vi "SVFA Power Spectrum (N Ch).vi"(0 "scaled signals [EU]":waveform(dbl)[](array[waveform]), 2 "window":T8=1 items=["None"=0, "Hanning"=1, "Hamming"=2, "Blackman-Harris"=3, "Exact Blackman"=4, "Blackman"=5, "Flat Top"=6, "4 Term B-Harris "=7, "7 Term B-Harris"=8, "Low Sidelobe"=9, "Force"=64, "Exponential"=65, "Blackman Nuttall"=11, "Triangle"=30, "Bartlett-Hanning"=31, "Bohman"=32, "Parzen"=33, "Welch"=34, "Kaiser"=60, "Dolph-Chebyshev"=61, "Gaussian"=62], 4 "dB On (T)":bool=TRUE, 5 "error in (no error)":errorcluster, 7 "averaging parameters":T7={"averaging mode"=enum."No averaging", "weighting mode"=enum."Exponential", "number of averages"=10, "linear mode"=enum."One shot"}, 9 "restart averaging (F)":bool) -> (11 "averaging done":bool, 13 "averages completed":dbl, 14 "power spectra [dB EU]":cluster{"f0":dbl, "df":dbl, "magnitude":dbl[]}[](array[cluster]) {"magnitude" format="%.2p"; "df" format="%.2p"; "f0" format="%.2p"}, 15 "unit labels":string[](array[string]), 18 "spectrum info":T1[](array[typedef]) {"x-axis units" items=["Time (s)"=0, "Frequency-CB (Hz)"=1, "Frequency-CPB (Hz)"=1248, "Frequency-Arbitrary (Hz)"=2357, "Quefrency (s)"=2, "Revolutions (rev)"=3, "Order"=4, "Speed (RPM)"=11, "Speed (rad/s)"=21, "Index"=65535]; "weighting filter" items=["Linear", "A-weighting", "B-weighting", "C-weighting", "ITU-R 468-4", "Dolby", "CCITT", "C-message", "Wb", "Wc", "Wd", "We", "Wf", "Wh", "Wj", "Wk", "Wm", "AES17 20 kHz lowpass", "AES17 40 kHz lowpass", "AES17 20 kHz highpass", "AES17 40 kHz highpass"]; "dB reference [EU]" format="%.2f"; "engineering units" items=["custom..."=0, "V"=1, "A"=21, "C"=30, "pC"=31, "s"=32, "-"=29, "Pa"=2, "N"=20, "g"=3, "m/s^2"=4, "m/s"=5, "m"=6, "mm/s"=12, "mm"=13, "micron/s"=14, "micron"=15, "in/s^2"=7, "in/s"=8, "in"=9, "mil/s"=10, "mil"=11, "rad/s^2"=16, "rad/s"=17, "rad"=18, "deg/s^2"=26, "deg/s"=27, "deg"=28, "RPM"=22, "cycle/s^2"=23, "Hz"=24, "cycle"=25, "strain"=19]; "spectral info"."window" items=["None "=0, "Hanning"=1, "Hamming"=2, "Blackman-Harris"=3, "Exact Blackman"=4, "Blackman"=5, "Flat Top"=6, "4 Term B-Harris "=7, "7 Term B-Harris"=8, "Low Sidelobe"=9, "Force - Exponential"=10, "Gaussian"=62]}, 19 "error out":errorcluster)   [LabVIEW 2017]
doc: "Computes the power spectrum of <B>scaled signal [EU]</B>. Use the power spectrum to quantify signal components as a function of frequency. Wire data to the <B>scaled signal [EU]</B> input to determine the polymorphic instance to use or manually select the instance."
uses:
  <vilib>/addons/_NISVFA/_Shared subVIs/Controls/svc_Window.ctl
  <vilib>/addons/_NISVFA/_Shared subVIs/Controls/svc_Spectrum Info.ctl
  <vilib>/addons/_NISVFA/_Shared subVIs/Controls/svc_X-Axis Units.ctl
  <vilib>/addons/_NISVFA/_Shared subVIs/Controls/svc_Spectrum Type.ctl
  <vilib>/addons/_NISVFA/_Shared subVIs/Controls/svc_Engineering Units Text Ring.ctl
  <vilib>/addons/_NISVFA/_Shared subVIs/Controls/svc_Weighting Filter Text Ring.ctl
  <vilib>/addons/_NISVFA/_Shared subVIs/Controls/svc_Complimentary Spectrum Units.ctl
  <vilib>/Analysis/2dsp.llb/Power Spectrum (DBL).vi
  <vilib>/Analysis/2dsp.llb/Real FFT.vi
  <vilib>/addons/_NISVFA/_Shared subVIs/Spectrum Averaging/svfa_No Average Array (complex).vi
  <vilib>/Analysis/4window.llb/Force Window.vi
  <vilib>/Analysis/4window.llb/Force Window (DBL).vi
  <vilib>/Analysis/4window.llb/Exponential Window.vi
  <vilib>/Analysis/4window.llb/Exponential Window (DBL).vi
  <vilib>/addons/_NISVFA/_Shared subVIs/Common/svc_Get Weighting Enum and Labels.vi
  <vilib>/addons/_NISVFA/_Shared subVIs/Common/svc_Unit Label Lexical Class.vi
  <vilib>/addons/_NISVFA/_Shared subVIs/Common/svc_Engineering Units to Unit Label.vi
  <vilib>/addons/_NISVFA/_Shared subVIs/Common/svc_Format Value (DBL).vi
  <vilib>/Utility/error.llb/Error Cluster From Error Code.vi
  <vilib>/Analysis/0measdsp.llb/Scaled Time Domain Window.vi
  <vilib>/Analysis/0measdsp.llb/Scaled Time Domain Window (DBL).vi
  <vilib>/addons/_NISVFA/_Spectrum Processing/subVIs/svfa_Spectrum Info Window to windowTd Type Def.vi
  <vilib>/addons/_NISVFA/_Shared subVIs/Common/svc_Unit Label to Engineering Units.vi
  <vilib>/addons/_NISVFA/_Shared subVIs/Common/svc_Window Parameters.vi
  <vilib>/addons/_NISVFA/_Shared subVIs/Common/svc_Get Window Info.vi
  <vilib>/Analysis/NI_AALPro.lvlib
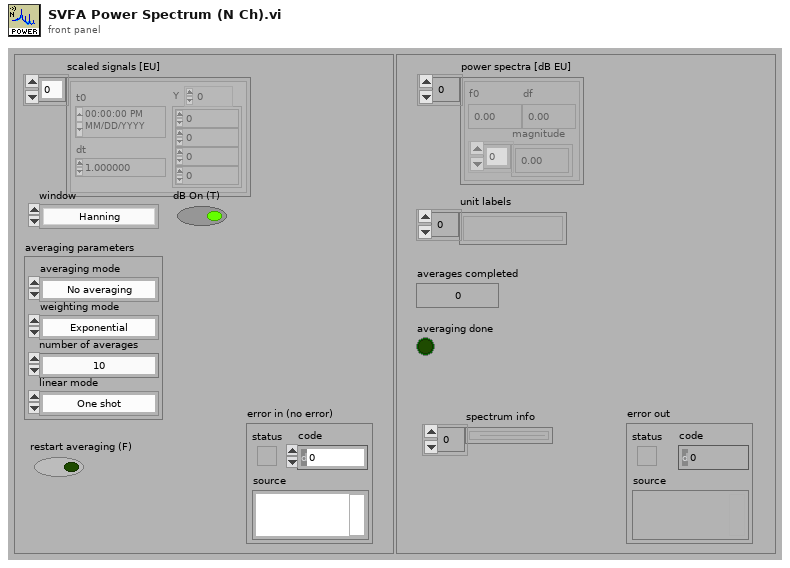
[diagram p1: front panel]
types:
  T1 = typedef "svc_Spectrum Info.ctl" = cluster{"channel name":string, "description":string, "x-axis units":T2, "spectral info":cluster{"spectrum type":T3, "linear/dB":enum16{"linear", "dB"}, "window":u16, "window size":i32, "FFT size":i32}, "engineering units":T4, "custom label":string, "dB reference [EU]":dbl, "peak units":enum16{"rms", "peak", "peak-peak"}, "weighting filter":T5, "spectral density?":bool, "unit label":string, "spectrum skewed?":bool, "complimentary spectrum units":T6}
  T2 = typedef "svc_X-Axis Units.ctl" = u16
  T3 = typedef "svc_Spectrum Type.ctl" = enum16{"FFT Spectrum [complex]", "Amplitude [Magnitude]", "Power [Magnitude^2]", "Cross Spectrum [complex]", "Frequency Response [Complex]"}
  T4 = typedef "svc_Engineering Units Text Ring.ctl" = u16
  T5 = typedef "svc_Weighting Filter Text Ring.ctl" = u16
  T6 = typedef "svc_Complimentary Spectrum Units.ctl" = enum16{"none", "radians", "degrees", "cycles", "imaginary"}
  T7 = cluster{"averaging mode":enum16{"No averaging", "Vector averaging", "RMS averaging", "Peak hold"}, "weighting mode":enum16{"Linear", "Exponential"}, "number of averages":u32, "linear mode":enum16{"One shot", "Auto restart"}}
  T8 = typedef "svc_Window.ctl" = u32
  T9 = enum16{"Restart processing", "Continue processing", "Skip processing"}
  T10 = cluster{"complex FFT":cdb[], "real FFT":dbl[], "f0":dbl, "df":dbl, "averages completed":dbl, "averaging parameters":cluster{"averaging mode":enum16{"No averaging", "Vector averaging", "RMS averaging", "Peak hold"}, "weighting mode":enum16{"Linear", "Exponential"}, "number of averages":u32, "linear mode":enum16{"One shot", "Auto restart"}}}
  T11 = cluster{"spectrum type":T3, "linear/dB":enum16{"linear", "dB"}, "window":u16, "window size":i32, "FFT size":i32}
  T12 = cluster{"complex FFT":cdb[], "real FFT":dbl[], "f0":dbl, "df":dbl, "averages completed":dbl, "averaging parameters":cluster{"averaging mode":enum16{"No averaging", "Vector averaging", "RMS averaging", "Peak hold"}, "weighting mode":enum16{"Linear", "Exponential"}, "number of averages":u32, "linear mode":enum16{"One shot", "Auto restart"}}}[]
  T13 = cluster{"complex FFT":cdb[], "Mag/Real FFT":dbl[], "f0":dbl, "df":dbl, "averages completed":dbl, "averaging parameters":cluster{"averaging mode":enum16{"No averaging", "Vector averaging", "RMS averaging", "Peak hold"}, "weighting mode":enum16{"Linear", "Exponential"}, "number of averages":u32, "linear mode":enum16{"One shot", "Auto restart"}}}[]
  T14 = enum16{"No averaging", "Vector averaging", "RMS averaging", "Peak hold"}
  T15 = typedef "svc_Channel Info.ctl" = cluster{"sensor sensitivity":dbl, "engineering units":T4, "dB reference":dbl, "custom label":string, "weighting filter":T5, "pregain":dbl}
  T16 = cluster{"complex FFT":cdb[], "Mag/Real FFT":dbl[], "f0":dbl, "df":dbl, "averages completed":dbl, "averaging parameters":cluster{"averaging mode":enum16{"No averaging", "Vector averaging", "RMS averaging", "Peak hold"}, "weighting mode":enum16{"Linear", "Exponential"}, "number of averages":u32, "linear mode":enum16{"One shot", "Auto restart"}}}
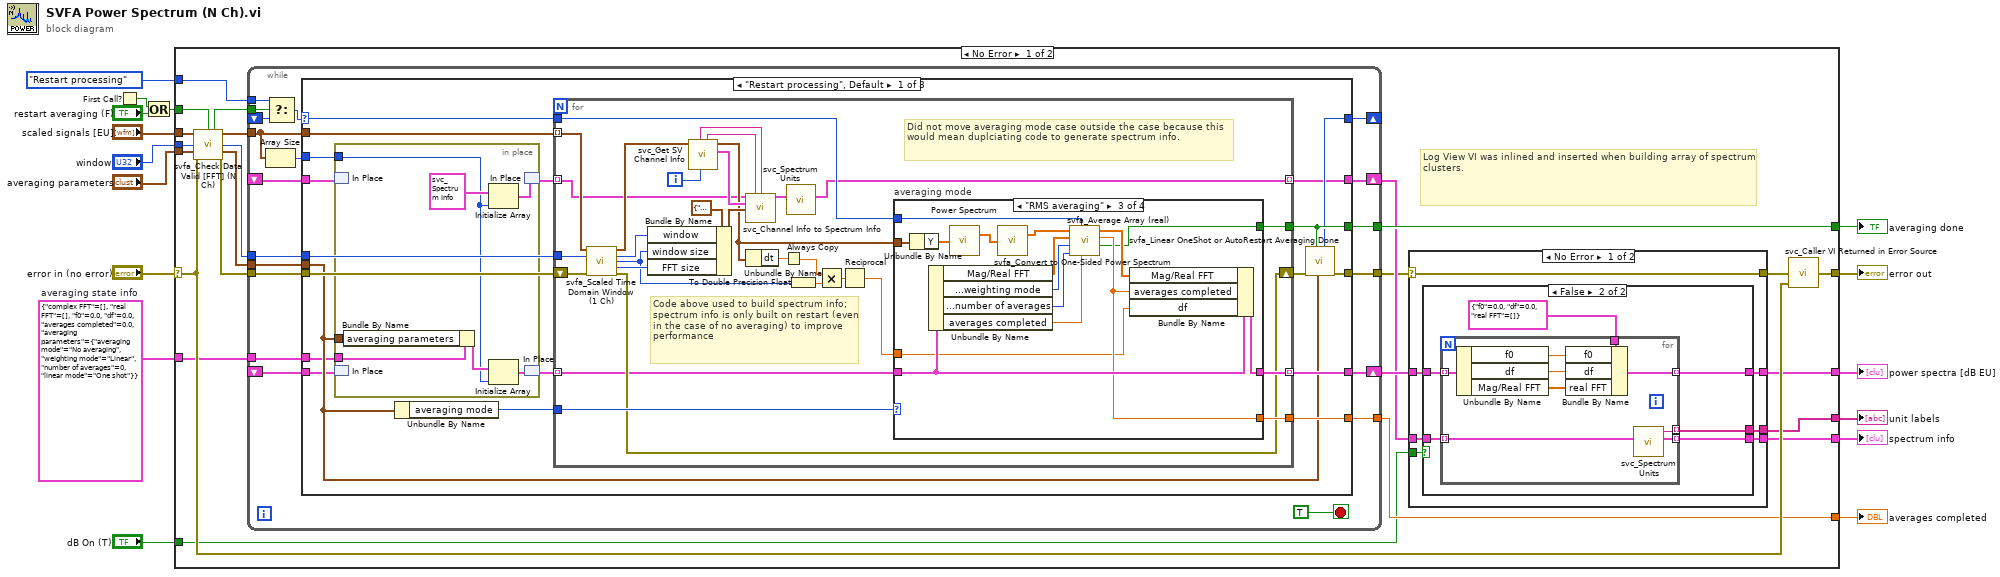
[diagram p0: block diagram]
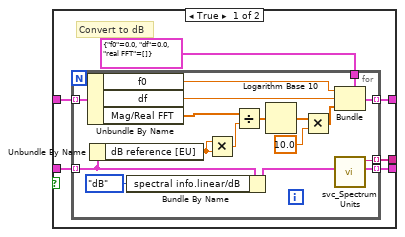
[diagram p2: hidden frame]
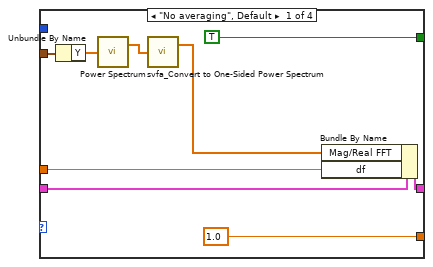
[diagram p4: hidden frame]
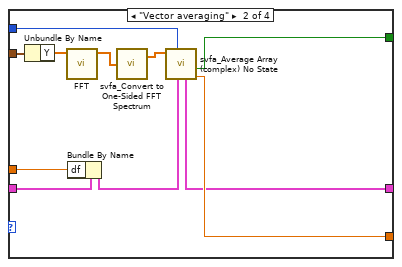
[diagram p5: hidden frame]
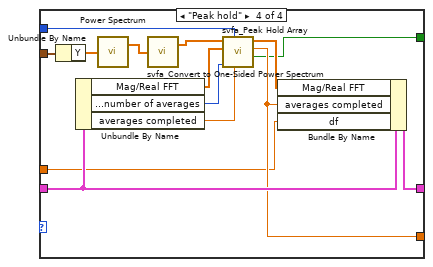
[diagram p6: hidden frame]
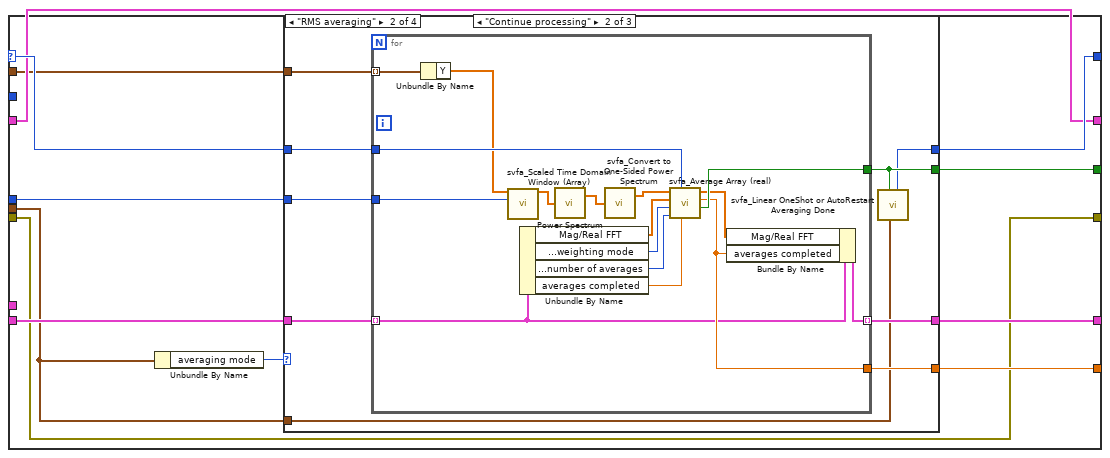
[diagram p7: hidden frame]
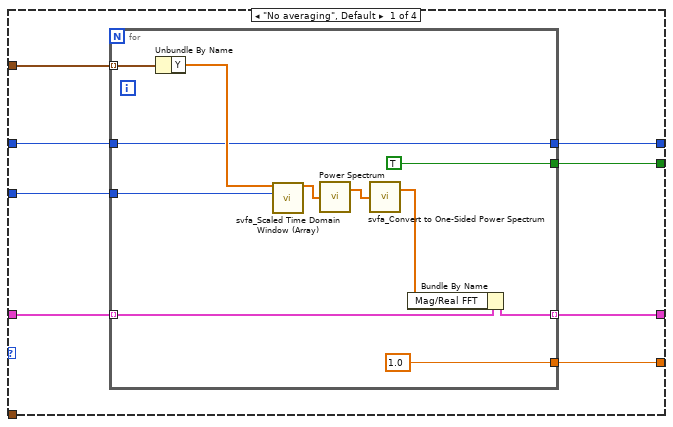
[diagram p8: hidden frame]
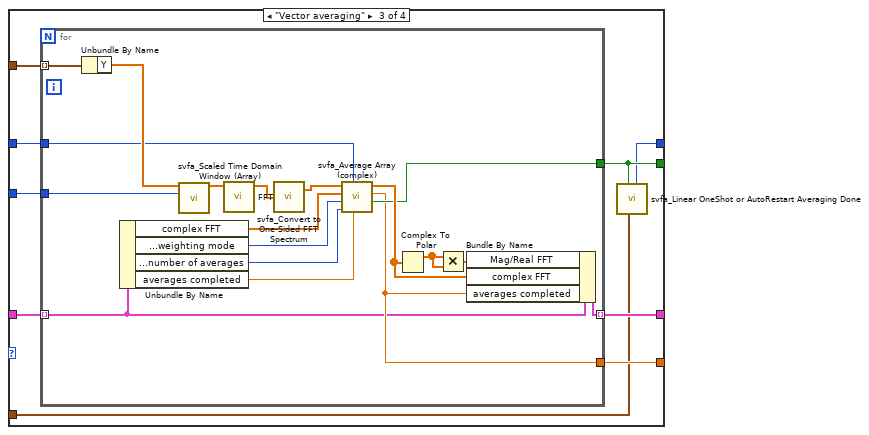
[diagram p9: hidden frame]
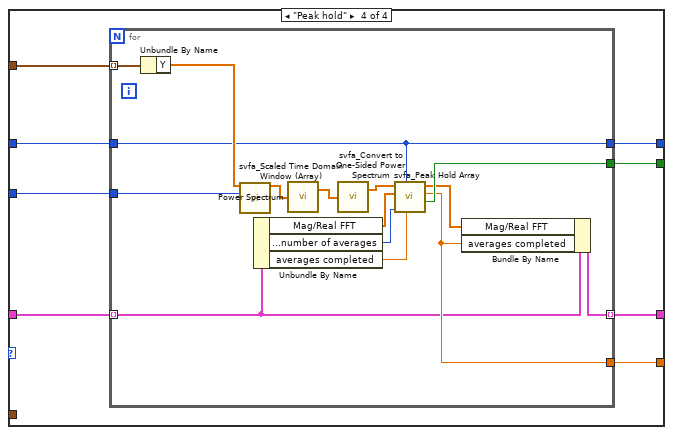
[diagram p10: hidden frame]
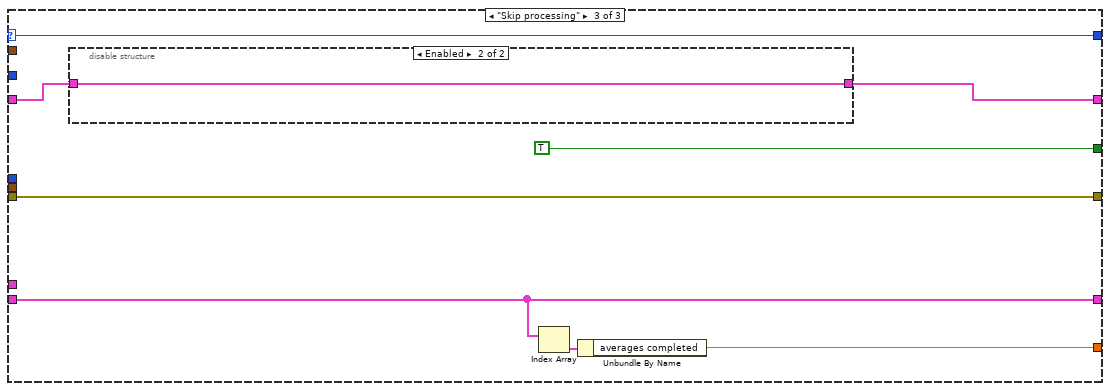
[diagram p11: hidden frame]
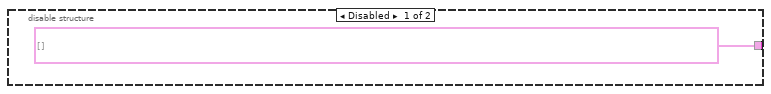
[diagram p12: hidden frame]
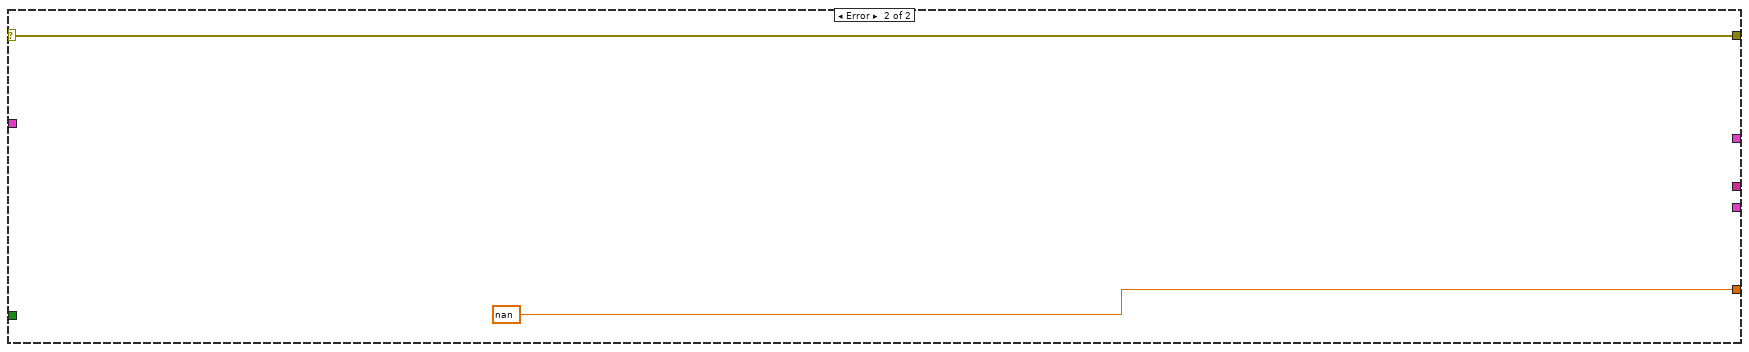
[diagram p13: hidden frame]
diagram:
  w2 = T10 {"complex FFT"=[], "real FFT"=[], "f0"=0.0, "df"=0.0, "averages completed"=0.0, "averaging parameters"={"averaging mode"=enum."No averaging", "weighting mode"=enum."Linear", "number of averages"=0, "linear mode"=enum."One shot"}}  # averaging state info
  n1 = First Call?() -> (First Call?: T/F=w8:bool)
  n2 = Or(x=w8, y="restart averaging (F)") -> (x .or. y?=w6:bool)
  n3 = case shown="No Error" "error in (no error)" {
    selector: "error in (no error)" -> [w34 w326]
    tunnel: "scaled signals [EU]" -> [w39 _]
    tunnel: w6 -> [w36 _]
    tunnel: [w35 w326] -> w15
    tunnel: [w21 _] -> w14
    tunnel: [w31 _] -> w13
    tunnel: [w32 nan ("averages completed")] -> w12
    tunnel: [w23 _] -> w11
    tunnel: "window" -> [w38 _]
    tunnel: "averaging parameters" -> [w37 _]
    tunnel: "dB On (T)" -> [w18 _]
    tunnel: [w22 _] -> w4
    tunnel: w2 -> [w25 _]
    tunnel: T9."Restart processing" ("t") -> [w17 _]
    frame No Error {
      # "Log View VI was inlined and inserted when building array of spectrum clusters."
      n4 = call <vilib>:"svfa_Check Data Valid [FFT] (N Ch).vi"("scaled signals"=w39, "restart averaging (F)"=w36, "window"=w38, "averaging parameters"=w37, "error in (no error)"=w34) -> ("restart averaging"=w28:bool, "dup scaled signals"=w27:waveform(dbl)[], "dup window"=w30:T8, "dup averaging parameters"=w33:T7, "error out"=w29:errorcluster)  [unwired: 6 in]
      n5 = while {
        tunnel: w30 -> [w98]
        tunnel: [w99] -> w32
        tunnel: [w100] -> w31
        tunnel: w33 -> [w101]
        tunnel: [w102] -> w20
        shift-left: _ -> [w89]
        shift-right: [w103] -> w26
        tunnel: w29 -> [w104]
        shift-right: [w97] -> w24
        shift-left: _ -> [w96]
        shift-right: [w95] -> _
        shift-left: _ -> [w94]
        tunnel: w28 -> [w92]
        tunnel: w17 -> [w91]
        tunnel: w25 -> [w90]
        tunnel: w27 -> [w88]
        stop <- TRUE stop-if-true
        n6 = Array Size(array=w88) -> (size(s)=w87:i32)
        n7 = Select(t=w91, s=w92, f=w94) -> (s? t:f=w93:T9)
        n8 = case shown="\"Restart processing\", Default" w93 {
          selector: w93 -> [w116 w218 w319]
          tunnel: w104 -> [w115 w210 w321]
          tunnel: w88 -> [w111 w211 _]
          tunnel: [w123 w221 w320] -> w103
          tunnel: w89 -> [w110 w217 w320]
          tunnel: [w118 w210 w321] -> w102
          tunnel: w101 -> [w113 w214 _]
          tunnel: [w121 w219 TRUE ("averaging done")] -> w100
          tunnel: [w122 w220 w322] -> w99
          tunnel: w98 -> [w117 w216 _]
          tunnel: [w114 w212 w317] -> w97
          tunnel: w96 -> [w107 w212 w316]
          tunnel: [w120 w213 w319] -> w95
          tunnel: w90 -> [w112 _ _]
          tunnel: w87 -> [w106 _ _]
          frame "Restart processing", Default {
            n9 = in-place {
              in-place-border: w113 -> [w131]
              in-place-border: w112 -> [w130]
              in-place-border: w106 -> [w125]
              n10 = in-place-match #1(w107) -> ()  [unwired: 1 out]
              n11 = in-place-match #2(w110) -> ()  [unwired: 1 out]
              n12 = Bundle By Name(cluster=w130, "averaging parameters"=w131) -> (w129:T10)
              n13 = Initialize Array(T1 {"channel name"="", "description"="", "x-axis units"=0, "spectral info"={"spectrum type"=enum."Power [Magnitude^2]", "linear/dB"=enum."linear", "window"=0, "window size"=0, "FFT size"=0}, "engineering units"=0, "custom label"="", "dB reference [EU]"=0.0, "peak units"=enum."rms", "weighting filter"=0, "spectral density?"=FALSE, "unit label"="", "spectrum skewed?"=FALSE, "complimentary spectrum units"=enum."none"} ("spectrum info out"), w125) -> (w126:T1[])
              n14 = Initialize Array(w129, w125) -> (w128:T12)
              n15 = in-place-match #1(w126) -> (w108:T1[])
              n16 = in-place-match #2(w128) -> (w109:T13)
            }
            n17 = Unbundle By Name(w113) -> ("averaging mode"=w124:T14)
            n18 = for {
              tunnel: [w159] -> w123 mode=indexing
              tunnel: [w158] -> w121
              tunnel: [w157] -> w122
              tunnel: w124 -> [w156]
              tunnel: w109 -> [w141] mode=indexing
              tunnel: w116 -> [w154]
              shift-right: [w143] -> w119
              shift-left: w115 -> [w153]
              tunnel: w117 -> [w155]
              tunnel: w108 -> [w132] mode=indexing
              tunnel: [w146] -> w114 mode=indexing
              tunnel: w111 -> [w134] mode=indexing
              i -> [w142]
              # "Did not move averaging mode case outside the case because this would mean duplciating code to generate spectrum info."
              # "Code above used to build spectrum info; spectrum info is only built on restart (even in the case of no averaging) to improve performance"
              n19 = call <vilib>:"svfa_Scaled Time Domain Window (1 Ch).vi"("Signal in [X]"=w134, "window"=w155, "error in"=w153) -> ("Windowed Waveform"=w147:waveform(dbl), "dup window"=w145:T8, "window length"=w137:i32, "FFT length"=w144:i32, "error out"=w143:errorcluster)  [unwired: 7 in, 1 out]
              n20 = Bundle By Name(cluster=T11 {"spectrum type"=enum."Power [Magnitude^2]", "linear/dB"=enum."linear", "window"=0, "window size"=0, "FFT size"=0} ("spectral info"), "window"=w145, "window size"=w137, "FFT size"=w144) -> (w151:T11)
              n21 = call <vilib>:"svc_Get SV Channel Info.vi"("channel index"=w142, "scaled signal [EU]"=w147) -> ("channel info"=w150:T15, "dup scaled signal [EU]"=w135:waveform(dbl), "channel name"=w148:string, "channel description"=w149:string)  [unwired: 4 in, 2 out]
              n22 = call <vilib>:"svc_Channel Info to Spectrum Info.vi"("spectrum info in"=w132, "channel name"=w148, "description"=w149, "channel info"=w150, "spectral info"=w151) -> ("spectrum info out"=w152:T1)  [unwired: 10 in]
              n23 = Unbundle By Name ("Get Waveform Components")(w135) -> ("dt"=w139:dbl)
              n24 = Always Copy(1:w139) -> (0:w136:dbl)
              n25 = call <vilib>:"svc_Spectrum Units.vi"("spectrum info in"=w152) -> ("spectrum info out"=w146:T1)  [unwired: 3 in, 3 out]
              n26 = To Double Precision Float(number=w137) -> (double precision float=w138:dbl)
              n27 = Multiply(x=w136, y=w138) -> (x*y=w160:dbl)
              n28 = Reciprocal(x=w160) -> (1/x=w140:dbl)
              n29 = case "averaging mode" shown="\"RMS averaging\"" w156 {
                tunnel: [1.0 ("averages completed") w179 w188 w200] -> w157
                tunnel: [TRUE ("averaging done") w175 w187 w199] -> w158
                tunnel: w154 -> [_ w180 w191 w208]
                tunnel: [w165 w176 w192 w204] -> w159
                tunnel: w141 -> [w166 w173 w190 w205]
                tunnel: w140 -> [w163 w172 w183 w198]
                tunnel: w135 -> [w162 w171 w182 w197]
                frame "No averaging", Default {
                  n30 = Unbundle By Name ("Get Waveform Components")(w162) -> ("Y"=w161:dbl[])
                  n31 = call-poly <vilib>:"Power Spectrum.vi"("X"=w161) -> ("Power Spectrum"=w167:dbl[])  [unwired: 1 out]
                  n32 = call <vilib>:"svfa_Convert to One-Sided Power Spectrum.vi"("two-sided power spectrum"=w167) -> ("one-sided power spectrum"=w164:dbl[])  [unwired: 1 out]
                  n33 = Bundle By Name(cluster=w166, "Mag/Real FFT"=w164, "df"=w163) -> (w165:T16)
                }
                frame "Vector averaging" {
                  n34 = Unbundle By Name ("Get Waveform Components")(w171) -> ("Y"=w170:dbl[])
                  n35 = call-poly <vilib>:"FFT.vi"("X"=w170) -> ("FFT {X}"=w178:cdb[])  [unwired: 9 in, 1 out]
                  n36 = Bundle By Name(cluster=w173, "df"=w172) -> (w174:T16)
                  n37 = call <vilib>:"svfa_Convert to One-Sided FFT Spectrum.vi"("two-sided FFT spectrum"=w178) -> ("one-sided FFT spectrum"=w177:cdb[])  [unwired: 1 out]
                  n38 = call <vilib>:"svfa_Average Array (complex) No State.vi"("averaging state info in"=w174, "processing control"=w180, "array"=w177) -> ("averages completed"=w179:dbl, "averaging done"=w175:bool, "averaging state info out"=w176:T16)  [unwired: 5 in, 1 out]
                }
                frame "RMS averaging" {
                  n39 = Unbundle By Name ("Get Waveform Components")(w182) -> ("Y"=w181:dbl[])
                  n40 = Unbundle By Name(w190) -> ("Mag/Real FFT"=w193:dbl[], "averaging parameters.weighting mode"=w186:enum16{"Linear", "Exponential"}, "averaging parameters.number of averages"=w185:u32, "averages completed"=w184:dbl)
                  n41 = call-poly <vilib>:"Power Spectrum.vi"("X"=w181) -> ("Power Spectrum"=w195:dbl[])  [unwired: 1 out]
                  n42 = call <vilib>:"svfa_Convert to One-Sided Power Spectrum.vi"("two-sided power spectrum"=w195) -> ("one-sided power spectrum"=w194:dbl[])  [unwired: 1 out]
                  n43 = call <vilib>:"svfa_Average Array (real).vi"("averages completed in"=w184, "processing control"=w191, "number of averages"=w185, "weighting mode"=w186, "previous average array"=w193, "array"=w194) -> ("averaging done"=w187:bool, "averages completed out"=w188:dbl, "average array"=w189:dbl[])  [unwired: 3 in]
                  n44 = Bundle By Name(cluster=w190, "Mag/Real FFT"=w189, "averages completed"=w188, "df"=w183) -> (w192:T16)
                }
                frame "Peak hold" {
                  n45 = Unbundle By Name ("Get Waveform Components")(w197) -> ("Y"=w196:dbl[])
                  n46 = Unbundle By Name(w205) -> ("Mag/Real FFT"=w207:dbl[], "averaging parameters.number of averages"=w201:u32, "averages completed"=w202:dbl)
                  n47 = call-poly <vilib>:"Power Spectrum.vi"("X"=w196) -> ("Power Spectrum"=w209:dbl[])  [unwired: 1 out]
                  n48 = call <vilib>:"svfa_Convert to One-Sided Power Spectrum.vi"("two-sided power spectrum"=w209) -> ("one-sided power spectrum"=w206:dbl[])  [unwired: 1 out]
                  n49 = call <vilib>:"svfa_Peak Hold Array.vi"("averages completed in"=w202, "processing control"=w208, "number of averages"=w201, "previous peak array"=w207, "array"=w206) -> ("averaging done"=w199:bool, "averages completed out"=w200:dbl, "peak array"=w203:dbl[])  [unwired: 4 in]
                  n50 = Bundle By Name(cluster=w205, "Mag/Real FFT"=w203, "averages completed"=w200, "df"=w198) -> (w204:T16)
                }
              }
            }
            n51 = call <vilib>:"svfa_Linear OneShot or AutoRestart Averaging Done.vi"("averaging parameters"=w113, "averaging done"=w121, "error in (no error)"=w119) -> ("error out"=w118:errorcluster, "processing control"=w120:T9)  [unwired: 7 in]
          }
          frame "Continue processing" {
            # "This case should be as lean as possible for performance. One reason for using the lower-level averaging VIs was to manipulate the state cluster at the highest level to allow LV compiler to optimize memory copies. This added some complexity at the top level."
            n52 = Unbundle By Name(w214) -> ("averaging mode"=w215:T14)
            n53 = case "averaging mode" shown="\"RMS averaging\"" w215 {
              tunnel: [w229 w249 w274 w300] -> w221
              tunnel: [w228 w248 w273 w299] -> w220
              tunnel: [w227 w244 w269 w298] -> w219
              tunnel: w218 -> [w223 w247 w272 w295]
              tunnel: w217 -> [w226 w246 w271 w297]
              tunnel: w216 -> [w225 w245 w270 w296]
              tunnel: [w224 w243 w267 w293] -> w213
              tunnel: w214 -> [_ w242 w268 _]
              tunnel: w211 -> [w222 w241 w266 w294]
              frame "No averaging", Default {
                n54 = for {
                  tunnel: [w240] -> w229 mode=indexing
                  tunnel: [TRUE ("averaging done")] -> w227
                  tunnel: [1.0 ("averages completed")] -> w228
                  tunnel: w226 -> [w232] mode=indexing
                  tunnel: w225 -> [w235]
                  tunnel: [w231] -> w224
                  tunnel: w223 -> [w231]
                  tunnel: w222 -> [w230] mode=indexing
                  n55 = Unbundle By Name ("Get Waveform Components")(w230) -> ("Y"=w237:dbl[])
                  n56 = call <vilib>:"svfa_Scaled Time Domain Window (Array).vi"("input signal"=w237, "window"=w235) -> ("windowed signal"=w236:dbl[])  [unwired: 8 in, 5 out]
                  n57 = call-poly <vilib>:"Power Spectrum.vi"("X"=w236) -> ("Power Spectrum"=w234:dbl[])  [unwired: 1 out]
                  n58 = call <vilib>:"svfa_Convert to One-Sided Power Spectrum.vi"("two-sided power spectrum"=w234) -> ("one-sided power spectrum"=w233:dbl[])  [unwired: 1 out]
                  n59 = Bundle By Name(cluster=w232, "Mag/Real FFT"=w233) -> (w240:T16)
                }
              }
              frame "RMS averaging" {
                n60 = for {
                  tunnel: [w265] -> w249 mode=indexing
                  tunnel: [w263] -> w244
                  tunnel: [w262] -> w248
                  tunnel: w246 -> [w261] mode=indexing
                  tunnel: w247 -> [w264]
                  tunnel: w245 -> [w258]
                  tunnel: w241 -> [w250] mode=indexing
                  n61 = Unbundle By Name ("Get Waveform Components")(w250) -> ("Y"=w260:dbl[])
                  n62 = call <vilib>:"svfa_Scaled Time Domain Window (Array).vi"("input signal"=w260, "window"=w258) -> ("windowed signal"=w259:dbl[])  [unwired: 8 in, 5 out]
                  n63 = Unbundle By Name(w261) -> ("Mag/Real FFT"=w255:dbl[], "averaging parameters.weighting mode"=w253:enum16{"Linear", "Exponential"}, "averaging parameters.number of averages"=w252:u32, "averages completed"=w251:dbl)
                  n64 = call-poly <vilib>:"Power Spectrum.vi"("X"=w259) -> ("Power Spectrum"=w257:dbl[])  [unwired: 1 out]
                  n65 = call <vilib>:"svfa_Convert to One-Sided Power Spectrum.vi"("two-sided power spectrum"=w257) -> ("one-sided power spectrum"=w256:dbl[])  [unwired: 1 out]
                  n66 = call <vilib>:"svfa_Average Array (real).vi"("averages completed in"=w251, "processing control"=w264, "number of averages"=w252, "weighting mode"=w253, "previous average array"=w255, "array"=w256) -> ("averaging done"=w263:bool, "averages completed out"=w262:dbl, "average array"=w254:dbl[])  [unwired: 3 in]
                  n67 = Bundle By Name(cluster=w261, "Mag/Real FFT"=w254, "averages completed"=w262) -> (w265:T16)
                }
                n68 = call <vilib>:"svfa_Linear OneShot or AutoRestart Averaging Done.vi"("averaging parameters"=w242, "averaging done"=w244) -> ("processing control"=w243:T9)  [unwired: 8 in, 1 out]
              }
              frame "Vector averaging" {
                n69 = for {
                  tunnel: [w276] -> w274 mode=indexing
                  tunnel: [w279] -> w269
                  tunnel: [w278] -> w273
                  tunnel: w271 -> [w277] mode=indexing
                  tunnel: w272 -> [w281]
                  tunnel: w270 -> [w290]
                  tunnel: w266 -> [w275] mode=indexing
                  n70 = Unbundle By Name ("Get Waveform Components")(w275) -> ("Y"=w292:dbl[])
                  n71 = Unbundle By Name(w277) -> ("complex FFT"=w285:cdb[], "averaging parameters.weighting mode"=w287:enum16{"Linear", "Exponential"}, "averaging parameters.number of averages"=w286:u32, "averages completed"=w288:dbl)
                  n72 = call <vilib>:"svfa_Scaled Time Domain Window (Array).vi"("input signal"=w292, "window"=w290) -> ("windowed signal"=w291:dbl[])  [unwired: 8 in, 5 out]
                  n73 = call-poly <vilib>:"FFT.vi"("X"=w291) -> ("FFT {X}"=w289:cdb[])  [unwired: 9 in, 1 out]
                  n74 = call <vilib>:"svfa_Convert to One-Sided FFT Spectrum.vi"("two-sided FFT spectrum"=w289) -> ("one-sided FFT spectrum"=w280:cdb[])  [unwired: 1 out]
                  n75 = call <vilib>:"svfa_Average Array (complex).vi"("averages completed in"=w288, "processing control"=w281, "number of averages"=w286, "weighting mode"=w287, "previous average array"=w285, "array"=w280) -> ("averaging done"=w279:bool, "averages completed out"=w278:dbl, "average array"=w283:cdb[])  [unwired: 3 in]
                  n76 = Complex To Polar(r * e^(i*theta)=w283) -> (r=w284:dbl[])  [unwired: 1 out]
                  n77 = Multiply(x=w284, y=w284) -> (x*y=w282:dbl[])
                  n78 = Bundle By Name(cluster=w277, "Mag/Real FFT"=w282, "complex FFT"=w283, "averages completed"=w278) -> (w276:T16)
                }
                n79 = call <vilib>:"svfa_Linear OneShot or AutoRestart Averaging Done.vi"("averaging parameters"=w268, "averaging done"=w269) -> ("processing control"=w267:T9)  [unwired: 8 in, 1 out]
              }
              frame "Peak hold" {
                n80 = for {
                  tunnel: [w315] -> w300 mode=indexing
                  tunnel: [w314] -> w298
                  tunnel: [w313] -> w299
                  tunnel: w297 -> [w303] mode=indexing
                  tunnel: w295 -> [w302]
                  tunnel: w296 -> [w310]
                  tunnel: [w302] -> w293
                  tunnel: w294 -> [w301] mode=indexing
                  n81 = Unbundle By Name ("Get Waveform Components")(w301) -> ("Y"=w312:dbl[])
                  n82 = call <vilib>:"svfa_Scaled Time Domain Window (Array).vi"("input signal"=w312, "window"=w310) -> ("windowed signal"=w311:dbl[])  [unwired: 8 in, 5 out]
                  n83 = Unbundle By Name(w303) -> ("Mag/Real FFT"=w308:dbl[], "averaging parameters.number of averages"=w304:u32, "averages completed"=w305:dbl)
                  n84 = call-poly <vilib>:"Power Spectrum.vi"("X"=w311) -> ("Power Spectrum"=w309:dbl[])  [unwired: 1 out]
                  n85 = call <vilib>:"svfa_Convert to One-Sided Power Spectrum.vi"("two-sided power spectrum"=w309) -> ("one-sided power spectrum"=w307:dbl[])  [unwired: 1 out]
                  n86 = call <vilib>:"svfa_Peak Hold Array.vi"("averages completed in"=w305, "processing control"=w302, "number of averages"=w304, "previous peak array"=w308, "array"=w307) -> ("averaging done"=w314:bool, "averages completed out"=w313:dbl, "peak array"=w306:dbl[])  [unwired: 4 in]
                  n87 = Bundle By Name(cluster=w303, "Mag/Real FFT"=w306, "averages completed"=w313) -> (w315:T16)
                }
              }
            }
          }
          frame "Skip processing" {
            n88 = disable-structure shown="Enabled" {
              disable-tunnel: [T1[] [] ("f") w325] -> w317
              disable-tunnel: w316 -> [_ w325]
              frame Disabled {
              }
              frame Enabled {
              }
            }
            n89 = Index Array(array=w320) -> (element=w323:T16)  [unwired: 1 in]
            n90 = Unbundle By Name(w323) -> ("averages completed"=w322:dbl)
          }
        }
      }
      n91 = case shown="No Error" w20 {
        selector: w20 -> [w41 w86]
        tunnel: w26 -> [w46 _]
        tunnel: w24 -> [w45 w85]
        tunnel: [w44 _] -> w23
        tunnel: [w43 w85] -> w22
        tunnel: [w42 _] -> w21
        tunnel: [w41 w86] -> w19
        tunnel: w18 -> [w40 _]
        frame No Error {
          n92 = case shown="False" w40 {
            tunnel: w46 -> [w52 w75]
            tunnel: w45 -> [w50 w73]
            tunnel: [w49 w72] -> w44
            tunnel: [w48 w71] -> w43
            tunnel: [w47 w70] -> w42
            frame True {
              # "Convert to dB"
              n93 = for {
                tunnel: w52 -> [w67] mode=indexing
                tunnel: [w66] -> w47 mode=indexing
                tunnel: cluster{"f0":dbl, "df":dbl, "real FFT":dbl[]} {"f0"=0.0, "df"=0.0, "real FFT"=[]} ("cluster") -> [w65]
                tunnel: w50 -> [w60] mode=indexing
                tunnel: [w63] -> w48 mode=indexing
                tunnel: [w62] -> w49 mode=indexing
                n94 = Unbundle By Name(w67) -> ("f0"=w69:dbl, "df"=w68:dbl, "Mag/Real FFT"=w54:dbl[])
                n95 = Unbundle By Name(w60) -> ("dB reference [EU]"=w59:dbl)
                n96 = Bundle By Name(cluster=w60, "spectral info.linear/dB"=enum16{"linear", "dB"}."dB" ("Spectral Info.linear/dB")) -> (w61:T1)
                n97 = Multiply(x=w59, y=w59) -> (x*y=w55:dbl)
                n98 = Divide(x=w54, y=w55) -> (x/y=w58:dbl[])
                n99 = Logarithm Base 10(1:w58) -> (0:w57:dbl[])
                n100 = Multiply(x=w57, y=10.0) -> (x*y=w53:dbl[])
                n101 = Bundle(cluster=w65, "f0"=w69, "df"=w68, "real FFT"=w53) -> (w66:cluster{"f0":dbl, "df":dbl, "real FFT":dbl[]})
                n102 = call <vilib>:"svc_Spectrum Units.vi"("spectrum info in"=w61) -> ("spectrum info out"=w63:T1, "unit label"=w62:string)  [unwired: 3 in, 2 out]
              }
            }
            frame False {
              n103 = for {
                tunnel: w75 -> [w82] mode=indexing
                tunnel: [w81] -> w70 mode=indexing
                tunnel: cluster{"f0":dbl, "df":dbl, "real FFT":dbl[]} {"f0"=0.0, "df"=0.0, "real FFT"=[]} ("cluster") -> [w80]
                tunnel: w73 -> [w76] mode=indexing
                tunnel: [w79] -> w71 mode=indexing
                tunnel: [w78] -> w72 mode=indexing
                n104 = Unbundle By Name(w82) -> ("f0"=w84:dbl, "df"=w83:dbl, "Mag/Real FFT"=w77:dbl[])
                n105 = Bundle By Name(cluster=w80, "f0"=w84, "df"=w83, "real FFT"=w77) -> (w81:cluster{"f0":dbl, "df":dbl, "real FFT":dbl[]})
                n106 = call <vilib>:"svc_Spectrum Units.vi"("spectrum info in"=w76) -> ("spectrum info out"=w79:T1, "unit label"=w78:string)  [unwired: 3 in, 2 out]
              }
            }
          }
        }
        frame Error {
          # "Clear results in error case to make sure that users cannot use an invalid result. Pass spectrum info in case that can give clue as to which input parameter is invalid"
        }
      }
      n107 = call <vilib>:"svc_Caller VI Returned in Error Source.vi"("warning input to caller"=w34, "error in (no error)"=w19) -> ("error out"=w35:errorcluster)  [unwired: 3 in]
    }
    frame Error {
    }
  }
  "error out" <- w15
  "averaging done" <- w13
  "averages completed" <- w12
  "unit labels" <- w11
  "power spectra [dB EU]" <- w14
  "spectrum info" <- w4
